vi "CRYMake Frequency Array to Resolution.vi"(6 "dz(Hz)":dbl, 8 "Fs":dbl, 9 "Resolution":u16, 10 "Stop Freq":dbl, 11 "Start Freq":dbl) -> (3 "Frequency Array":dbl[](array[numeric]))   [LabVIEW 2013]
uses:
  Stimulus/SubVI/CRYStimulus Global.vi
panel:
  out "10^x":dbl
  out "2^x":dbl
  in  "Step Resolution1":u16(ring) caption="Resolution" items=["R10(1/3 Oct.)", "R20(1/6 Oct.)", "R40(1/12 Oct.)", "R80(1/24 Oct.)", "User Defined, Log", "User Defined,Linear"]
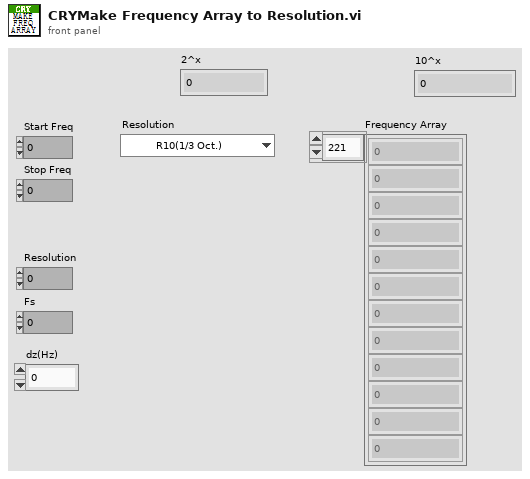
[diagram p1: front panel]
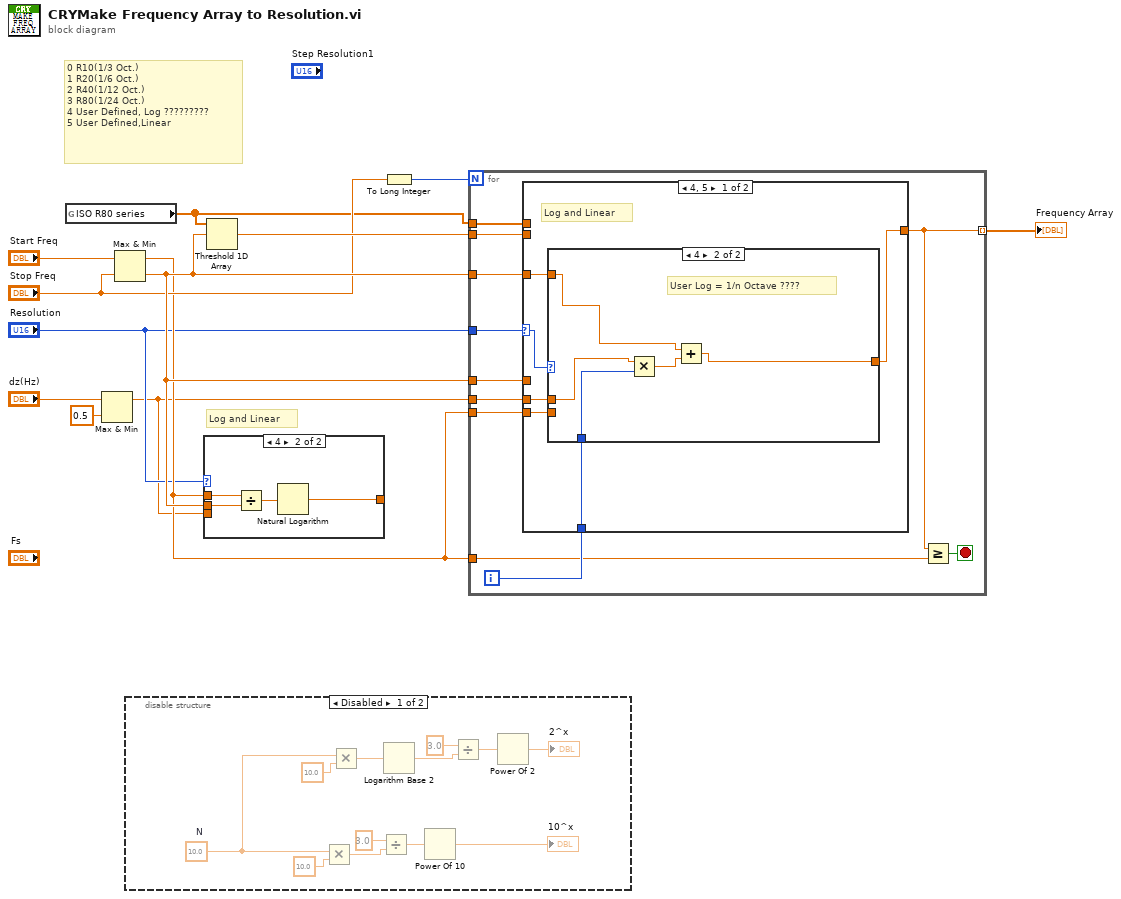
[diagram p0: block diagram]
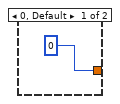
[diagram p3: hidden frame]
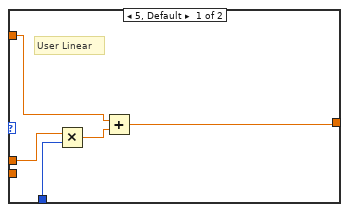
[diagram p4: hidden frame]
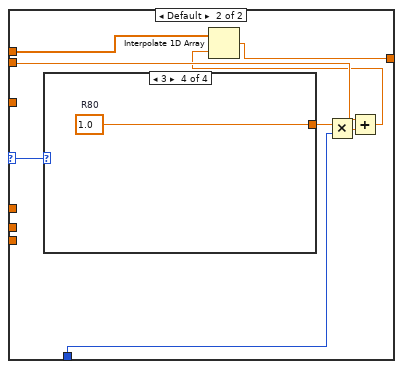
[diagram p5: hidden frame]
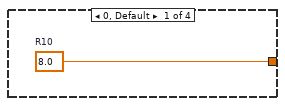
[diagram p6: hidden frame]
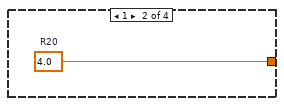
[diagram p7: hidden frame]
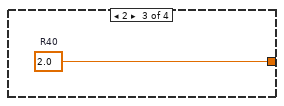
[diagram p8: hidden frame]
diagram:
  # "0 R10(1/3 Oct.)\n1 R20(1/6 Oct.)\n2 R40(1/12 Oct.)\n3 R80(1/24 Oct.)\n4 User Defined, Log ?????????\n5 User Defined,Linear"
  # "Log and Linear"
  n1 = global read "CRYStimulus Global.vi" "ISO R80 series"() -> (w1:dbl[])
  n2 = Max & Min(x="dz(Hz)", y=0.5) -> (max(x,y)=w2:dbl)  [unwired: 1 out]
  n3 = Max & Min(x="Start Freq", y="Stop Freq") -> (max(x,y)=w4:dbl, min(x,y)=w11:dbl)
  n4 = disable-structure shown="Disabled" {
    frame Disabled {
      w14 = 10.0  # N
      n5 = Multiply(x=w14, y=10.0 ("max(x,y)")) -> (x*y=w15:dbl)
      n6 = Multiply(x=w14, y=10.0 ("max(x,y)")) -> (x*y=w22:dbl)
      n7 = Divide(x=3.0 ("max(x,y)"), y=w15) -> (x/y=w17:dbl)
      n8 = Logarithm Base 2(1:w22) -> (0:w21:dbl)
      n9 = Power Of 10(x=w17) -> (10^x=→"10^x":dbl)
      n10 = Divide(x=3.0 ("max(x,y)"), y=w21) -> (x/y=w20:dbl)
      n11 = Power Of 2(x=w20) -> (2^x=→"2^x":dbl)
    }
    frame Enabled {
    }
  }
  n12 = case shown="4" "Resolution" {
    tunnel: w11 -> [_ w29]
    tunnel: w4 -> [_ w28]
    tunnel: [u16 0 ("Resolution") w26] -> _
    tunnel: w2 -> [_ _]
    frame 0, Default {
    }
    frame 4 {
      n13 = Divide(x=w28, y=w29) -> (x/y=w27:dbl)
      n14 = Natural Logarithm(1:w27) -> (0:w26:dbl)
    }
  }
  n15 = Threshold 1D Array(2:w11, 3:w1) -> (0:w12:dbl)  [unwired: 1 out]
  n16 = To Long Integer(number="Stop Freq") -> (32bit integer=w9:i32)
  n17 = for {
    N: w9 -> [_]
    tunnel: w12 -> [w40]
    tunnel: "Resolution" -> [w37]
    tunnel: w4 -> [w32]
    tunnel: w1 -> [w38]
    tunnel: w11 -> [w36]
    tunnel: w2 -> [w34]
    tunnel: w11 -> [w35]
    tunnel: [w33] -> w10 mode=indexing
    tunnel: w4 -> [w30]
    i -> [w39]
    stop <- w31 stop-if-true
    n18 = case shown="4, 5" w37 {
      selector: w37 -> [w43 w57]
      tunnel: w40 -> [_ w64]
      tunnel: w39 -> [w45 w60]
      tunnel: [w46 w59] -> w33
      tunnel: w38 -> [_ w58]
      tunnel: w36 -> [w44 _]
      tunnel: w35 -> [_ _]
      tunnel: w34 -> [w41 _]
      tunnel: w30 -> [w42 _]
      frame 4, 5 {
        # "Log and Linear"
        n19 = case shown="4" w43 {
          tunnel: w42 -> [_ _]
          tunnel: w44 -> [w50 w55]
          tunnel: w45 -> [w49 w54]
          tunnel: [w47 w52] -> w46
          tunnel: w41 -> [w48 w53]
          frame 5, Default {
            # "User Linear"
            n20 = Multiply(x=w48, y=w49) -> (x*y=w51:dbl)
            n21 = Add(x=w50, y=w51) -> (x+y=w47:dbl)
          }
          frame 4 {
            # "User Log = 1/n Octave ????"
            n22 = Multiply(x=w53, y=w54) -> (x*y=w56:dbl)
            n23 = Add(x=w55, y=w56) -> (x+y=w52:dbl)
          }
        }
      }
      frame Default {
        n24 = case shown="3" w57 {
          tunnel: [w65 w66 w67 w68] -> w63
          frame 0, Default {
            w65 = 8.0  # R10
          }
          frame 1 {
            w66 = 4.0  # R20
          }
          frame 2 {
            w67 = 2.0  # R40
          }
          frame 3 {
            w68 = 1.0  # R80
          }
        }
        n25 = Multiply(x=w63, y=w60) -> (x*y=w62:dbl)
        n26 = Add(x=w64, y=w62) -> (x+y=w61:dbl)
        n27 = Interpolate 1D Array(1:w61, 2:w58) -> (0:w59:dbl)
      }
    }
    n28 = Greater Or Equal?(x=w33, y=w32) -> (x >= y?=w31:bool)
  }
  "Frequency Array" <- w10
